vi "Create CO Channels.vi"(8 "error in":errorcluster, 10 "Channel Data in":T3 {"Device Chan Total" max=32 step=1; "Thermocouple"."Temperature Units" items=["Celcius", "Fahrenheit", "Kelvin", "Rankine", "Volts"]; "Thermocouple"."Thermocouple Type" items=["J", "K", "T", "E", "N", "B", "R", "S", "Raw Voltage"]}, 11 "Device Configuration Data In":T1 {"Current Section Ref" format="%.0x"; "simTC Section Refs" format="%.0x"; "Voltage Section Ref" format="%.0x"; "Custom Device Ref" format="%.0x"}) -> (0 "error out":errorcluster, 2 "Channel Data Out":T3 {"Device Chan Total" max=32 step=1; "Thermocouple"."Temperature Units" items=["Celcius", "Fahrenheit", "Kelvin", "Rankine", "Volts"]; "Thermocouple"."Thermocouple Type" items=["J", "K", "T", "E", "N", "B", "R", "S", "Raw Voltage"]}, 3 "Device Configuration Data Out":T1 {"Current Section Ref" format="%.0x"; "simTC Section Refs" format="%.0x"; "Voltage Section Ref" format="%.0x"; "Custom Device Ref" format="%.0x"})   [LabVIEW 2011, in "Simulated Thermocouple Custom Device.lvlib"]
uses:
  Simulated Thermocouple Custom Device.lvlib
  New Channel Data.ctl
  TC Selector.ctl
  TC Unit Selector.ctl
  Device Config data.ctl
  <vilib>/NI Veristand/Custom Device API/Custom Device Item Ref.ctl
  <vilib>/NI Veristand/Custom Device API/Custom Device Channel.ctl
  <vilib>/NI Veristand/Custom Device API/Custom Device Channel Type.ctl
  simTC Global GUIDs.vi
  <vilib>/NI Veristand/Custom Device API/Set Item Property (Variant).vi
  <vilib>/NI Veristand/Custom Device API/Set Item Property (String).vi
  <vilib>/NI Veristand/Custom Device API/Custom Device API.lvlib
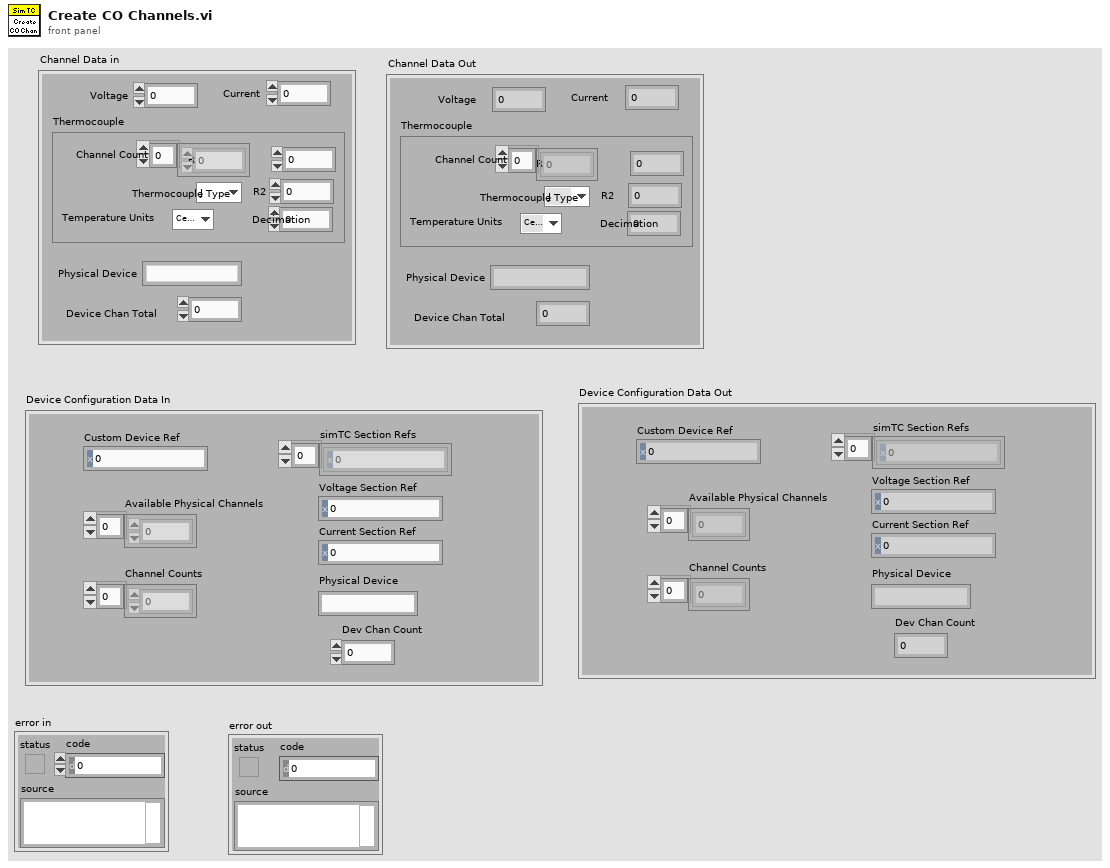
[diagram p1: front panel]
types:
  T1 = typedef "Simulated Thermocouple Custom Device.lvlib/Device Config data.ctl" = cluster{"Custom Device Ref":T2, "Voltage Section Ref":T2, "simTC Section Refs":T2[], "Current Section Ref":T2, "Physical Device":string, "Available Physical Channels":i32[], "Channel Counts":u32[], "Dev Chan Count":u32}
  T2 = typedef "Custom Device API.lvlib/Custom Device Item Ref.ctl" = u64
  T3 = typedef "Simulated Thermocouple Custom Device.lvlib/New Channel Data.ctl" = cluster{"Voltage":u32, "Current":u32, "Thermocouple":cluster{"R1":dbl, "R2":dbl, "Decimation":u32, "Thermocouple Type":T4, "Temperature Units":T5, "Channel Count":u32[]}, "Physical Device":string, "Device Chan Total":u32}
  T4 = typedef "Simulated Thermocouple Custom Device.lvlib/TC Selector.ctl" = u16
  T5 = typedef "Simulated Thermocouple Custom Device.lvlib/TC Unit Selector.ctl" = u16
  T6 = cluster{"Initial Value":dbl, "Range Min":dbl, "Range Max":dbl}
  T7 = typedef "Custom Device API.lvlib/Custom Device Channel.ctl" = cluster{"Type":T8, "Units":string, "Default Value":dbl, "Faultable":bool, "Scalable":bool}
  T8 = typedef "Custom Device API.lvlib/Custom Device Channel Type.ctl" = enum16{"Input", "Output"}
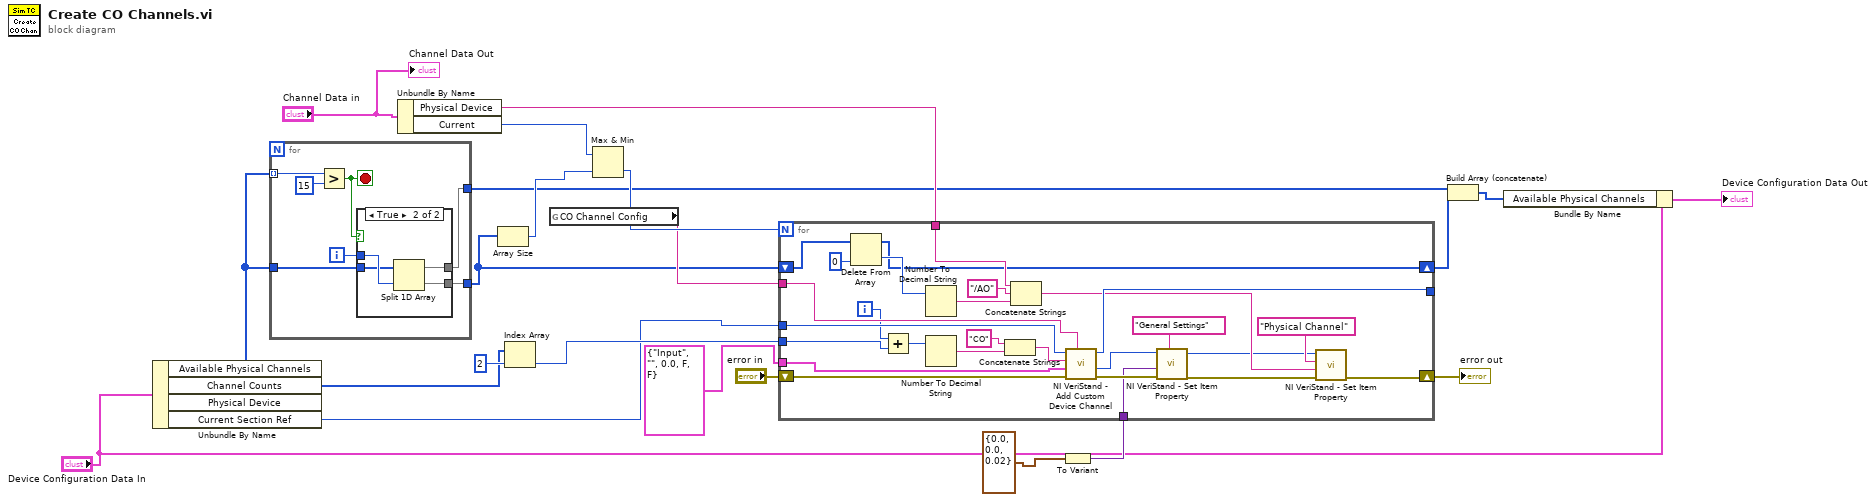
[diagram p0: block diagram]
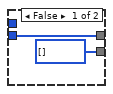
[diagram p2: hidden frame]
diagram:
  n1 = Unbundle By Name("Device Configuration Data In") -> ("Available Physical Channels"=w5:i32[], "Channel Counts"=w11:u32[], "Current Section Ref"=w12:T2)  [unwired: 1 out]
  n2 = for {
    tunnel: w5 -> [w28] mode=indexing
    tunnel: [w25] -> w4
    tunnel: [w24] -> w3
    tunnel: w5 -> [w23]
    i -> [w27]
    stop <- w26 stop-if-true
    n3 = Greater?(x=w28, y=15) -> (0:w26:bool)
    n4 = case shown="True" w26 {
      tunnel: w27 -> [_ w35]
      tunnel: [i32[] [] w34] -> w25
      tunnel: [w31 w33] -> w24
      tunnel: w23 -> [w31 w32]
      frame False {
      }
      frame True {
        n5 = Split 1D Array(array=w32, index=w35) -> (first subarray=w33:i32[], second subarray=w34:i32[])
      }
    }
  }
  n6 = Unbundle By Name("Channel Data in") -> ("Physical Device"=w10:string, "Current"=w15:u32)
  n7 = Array Size(array=w4) -> (size(s)=w16:i32)
  n8 = Index Array(array=w11, index=2) -> (element=w18:u32)
  n9 = global read "simTC Global GUIDs.vi" "CO Channel Config"() -> (w13:string)
  n10 = Max & Min(x=w15, y=w16) -> (min(x,y)=w17:u32)  [unwired: 1 out]
  n11 = To Variant(anything=T6 {"Initial Value"=0.0, "Range Min"=0.0, "Range Max"=0.02} ("CO Channel Config")) -> (Variant=w9:variant)
  n12 = for {
    N: w17 -> [_]
    tunnel: T7 {"Type"=enum."Input", "Units"="", "Default Value"=0.0, "Faultable"=FALSE, "Scalable"=FALSE} ("Channel") -> [w59]
    tunnel: w12 -> [w58]
    shift-right: [w38] -> w21
    shift-left: "error in" -> [w50]
    tunnel: [w57] -> _
    tunnel: w13 -> [w56]
    tunnel: w18 -> [w54]
    tunnel: w10 -> [w49]
    shift-right: [w47] -> w2
    shift-left: w4 -> [w37]
    tunnel: w9 -> [w45]
    i -> [w52]
    n13 = Delete From Array(array=w37, index=0) -> (deleted portion=w48:i32, array with subset deleted=w47:i32[])  [unwired: 1 in]
    n14 = Add(x=w52, y=w54) -> (x+y=w53:u32)
    n15 = Number To Decimal String(number=w48) -> (decimal integer string=w51:string)  [unwired: 1 in]
    n16 = Number To Decimal String(number=w53) -> (decimal integer string=w60:string)  [unwired: 1 in]
    n17 = Concatenate Strings("CO" ("Channel Name"), w60) -> (w62:string)
    n18 = Concatenate Strings(w49, "/AO", w51) -> (w40:string)
    n19 = call <vilib>:"NI VeriStand - Add Custom Device Channel.vi"("GUID (Default Channel)"=w56, "error in (no error)"=w50, "Channel"=w59, "Channel Name"=w62, "Parent Ref in"=w58) -> ("error out"=w46:errorcluster, "Channel Ref"=w43:T2, "Parent Ref out"=w57:T2)  [unwired: 3 in, 1 out]
    n20 = call-poly <vilib>:"NI VeriStand - Set Item Property.vi"("error in (no error)"=w46, "Value"=w45, "Property Name"="General Settings", "Item Ref in"=w43) -> ("error out"=w42:errorcluster, "Item Ref out"=w39:T2)  [unwired: 5 in, 1 out]
    n21 = call-poly <vilib>:"NI VeriStand - Set Item Property.vi"("error in (no error)"=w42, "Value"=w40, "Property Name"="Physical Channel", "Item Ref in"=w39) -> ("error out"=w38:errorcluster)  [unwired: 5 in, 2 out]
  }
  "error out" <- w21
  n22 = Build Array (concatenate)(w3, w2) -> (w1:i32[])
  n23 = Bundle By Name(cluster="Device Configuration Data In", "Available Physical Channels"=w1) -> (→"Device Configuration Data Out":T1)
  "Channel Data Out" <- "Channel Data in"
